vi "Mixer Launcher.vi"(9 "Sub Panel":refnum<vi>, 10 "Mixer ID":string="Secondary", 11 "Feeder Actor In":refnum<class "Feeder.lvclass">) -> (2 "Nested Actor's Enqueuer":refnum<class "Message Enqueuer.lvclass">, 3 "Feeder Actor Out":refnum<class "Feeder.lvclass">)   [LabVIEW 2018, in "Feeder Actor.lvlib" / "Mixer.lvclass"]
uses:
  Mixer.lvclass
  <vilib>/ActorFramework/Message Enqueuer/Message Enqueuer.lvclass
  Feeder/Feeder.lvclass
  C:/Program Files/National Instruments/LabVIEW 2018/vi.lib/MGI/Panel Manager/Panel Actor/Panel Actor/Panel Actor.lvclass
  Mixer.lvclass/Mixer.ctl
  <vilib>/MGI/Panel Manager/Panel/Panel/Subpanel/Subpanel.lvclass
  C:/Program Files/National Instruments/LabVIEW 2018/vi.lib/MGI/Panel Manager/Panel/Panel/Panel.lvclass
  <vilib>/DAQmx/create/channels.llb/DAQmx Create Channel (CO-Pulse Generation-Frequency).vi
  <vilib>/DAQmx/configure/timing.llb/DAQmx Timing (Implicit).vi
  <vilib>/MGI/Panel Manager/Panel/Panel/Subpanel/Subpanel.vi
  <vilib>/MGI/Panel Manager/Panel/Panel.lvlib
  <vilib>/MGI/Panel Manager/Panel Actor/Panel Actor/Panel Actor.lvclass
  ADM/Main.lvlib
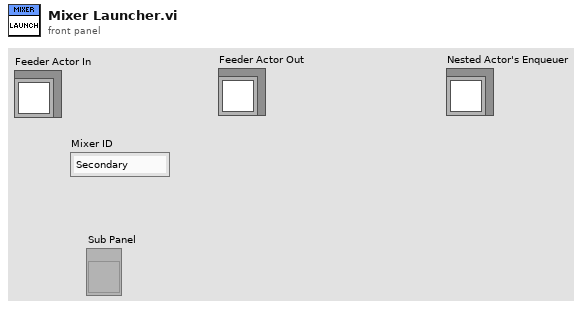
[diagram p1: front panel]
types:
  T1 = cluster{"Task Name":string, "Task Type":enum16{"VISA", "DAQmx"}, "VISA Resource Name":refnum<visa-resource-name>, "DAQmx Channel Name":tag}
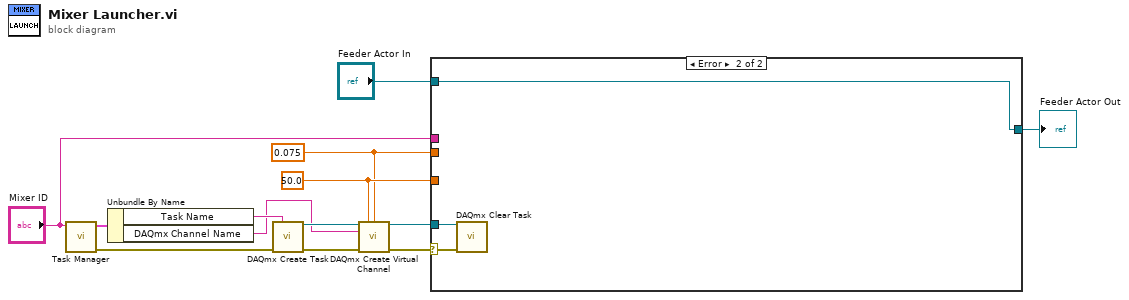
[diagram p0: block diagram]
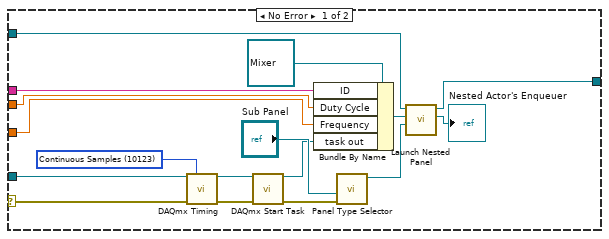
[diagram p2: hidden frame]
diagram:
  w10 = 0.075 ("duty cycle")
  w11 = 50.0 ("frequency")
  n1 = call "Task Manager.vi"("Task"="Mixer ID") -> ("error out"=w5:errorcluster, "Task Properties"=w4:T1)  [unwired: 9 in]
  n2 = Unbundle By Name(w4) -> ("Task Name"=w3:string, "DAQmx Channel Name"=w2:tag)
  n3 = call <vilib>:"DAQmx Create Task.vi"("new task name"=w3, "error in"=w5) -> ("task out"=w13:refnum<k21>, "error out"=w8:errorcluster)  [unwired: 12 in]
  n4 = call-poly <vilib>:"DAQmx Create Virtual Channel.vi"("task in"=w13, "frequency"=w11, "duty cycle"=w10, "counter"=w2, "error in"=w8) -> ("task out"=w12:refnum<k21>, "error out"=w9:errorcluster)  [unwired: 9 in]
  n5 = case shown="Error" w9 {
    selector: w9 -> [w16 w31]
    tunnel: "Feeder Actor In" -> [w29 w33]
    tunnel: [w28 w33] -> w6
    tunnel: "Mixer ID" -> [w21 _]
    tunnel: w12 -> [w19 w32]
    tunnel: w11 -> [w18 _]
    tunnel: w10 -> [w17 _]
    frame No Error {
      w22 = 10123 items=["Finite Samples"=10178, "Continuous Samples"=10123, "Hardware Timed Single Point"=12522] ("sample mode")
      n6 = call-poly <vilib>:"DAQmx Timing.vi"("task/channels in"=w19, "sample mode"=w22, "error in"=w16) -> ("task out"=w24:refnum<k21>, "error out"=w23:errorcluster)  [unwired: 11 in]
      n7 = call <vilib>:"DAQmx Start Task.vi"("task/channels in"=w24, "error in"=w23) -> ("task out"=w20:refnum<k21>, "error out"=w14:errorcluster)  [unwired: 12 in]
      n8 = Bundle By Name(cluster=refnum<class "Mixer.lvclass"> refnum ("Feeder Actor.lvlib:Mixer.lvclass"), "ID"=w21, "Duty Cycle"=w17, "Frequency"=w18, "task out"=w20) -> (w26:refnum<class "Mixer.lvclass">)
      n9 = call-poly <vilib>:"Panel Type Selector.vi"("Error In"=w14, "Sub Panel"="Sub Panel") -> ("Subpanel Out"=w27:refnum<class "Subpanel.lvclass">)  [unwired: 8 in, 1 out]
      n10 = call <vilib>:"Launch Nested Panel.vi"("Panel"=w27, "Nested Panel Actor"=w26, "Panel Actor in"=w29) -> ("Nested Actor's Enqueuer"=→"Nested Actor's Enqueuer":refnum<class "Message Enqueuer.lvclass">, "Panel Actor out"=w28:refnum<class "Feeder.lvclass">)  [unwired: 5 in, 2 out]
    }
    frame Error {
      n11 = call <vilib>:"DAQmx Clear Task.vi"("task in"=w32, "error in"=w31) -> ()  [unwired: 13 in, 1 out]
    }
  }
  "Feeder Actor Out" <- w6
